vi "InstallerBuildSpec.CommandLineArgs.vi"(8 "error in (no error)":errorcluster, 10 "New Version Command Line Argument":string, 11 "InstallerMutationSession":T1={"Installer Build Specification Ref"=refnum, "Project reference out"=refnum, "Installer Project Path"=path "C:/Users/Public/Documents/Git-Source/VeriStand-Custom-Steps-For-TestStand/Source/LabVIEW Code/Installer/Installer - Copy.lvproj"}) -> (0 "error out":errorcluster, 3 "InstallerMutationSession out":T1={"Installer Build Specification Ref"=refnum, "Project reference out"=refnum, "Installer Project Path"=path "C:/Users/Public/Documents/Git-Source/VeriStand-Custom-Steps-For-TestStand/Source/LabVIEW Code/Installer/Installer - Copy.lvproj"})   [LabVIEW 2013, in "VeriStand Steps Version Mutation.lvlib"]
uses:
  VeriStand Steps Version Mutation.lvlib
  Types/LVInstallerMutationSession.ctl
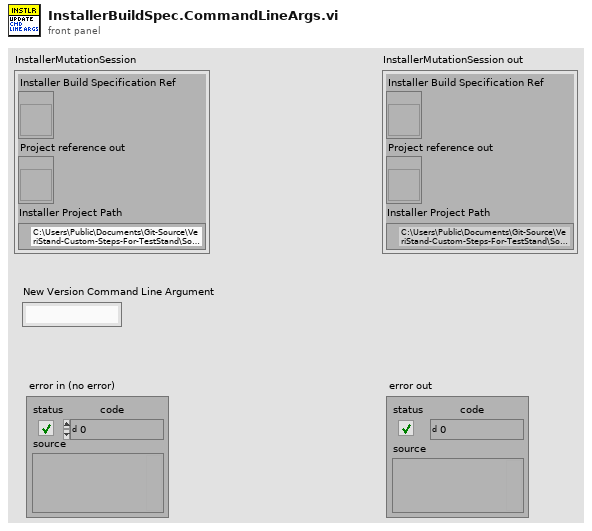
[diagram p1: front panel]
types:
  T1 = typedef "VeriStand Steps Version Mutation.lvlib/LVInstallerMutationSession.ctl" = cluster{"Installer Build Specification Ref":refnum<vi>, "Project reference out":refnum<vi>, "Installer Project Path":path}
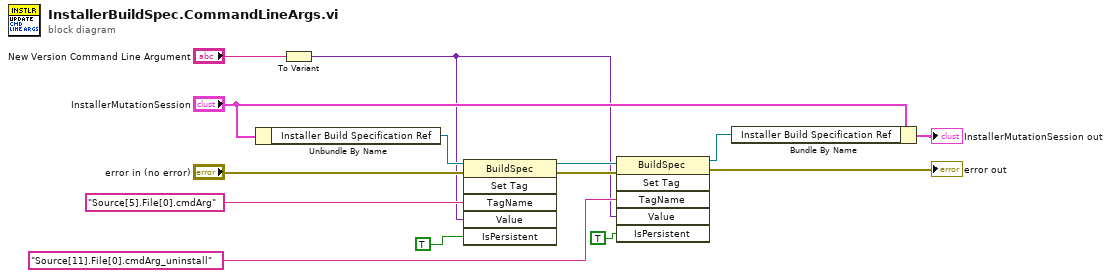
[diagram p0: block diagram]
diagram:
  n1 = Unbundle By Name("InstallerMutationSession") -> ("Installer Build Specification Ref"=w10:refnum<vi>)
  n2 = To Variant(anything="New Version Command Line Argument") -> (Variant=w4:variant)
  n3 = invoke class="BuildSpec" method="Set Tag"(reference=w10, error in="error in (no error)", "TagName"="Source[5].File[0].cmdArg" ("Tag Name"), "Value"=w4, "IsPersistent"=TRUE ("Is Persistent")) -> (reference out=w7:refnum<vi>, error out=w6:errorcluster)  [unwired: 1 in, 4 out]
  n4 = invoke class="BuildSpec" method="Set Tag"(reference=w7, error in=w6, "TagName"="Source[11].File[0].cmdArg_uninstall" ("Tag Name"), "Value"=w4, "IsPersistent"=TRUE ("Is Persistent")) -> (reference out=w2:refnum<vi>, error out=→"error out":errorcluster)  [unwired: 1 in, 4 out]
  n5 = Bundle By Name(cluster="InstallerMutationSession", "Installer Build Specification Ref"=w2) -> (→"InstallerMutationSession out":T1)
